vi "ZLIB Inflate__ogtk.vi"(4 "error in (no error)":errorcluster, 6 "expected length (try out)":i32, 7 "input":string) -> (0 "error out":errorcluster, 2 "length":i32, 3 "inflated output":string)   [LabVIEW 2014]
doc: "Inflates data previously deflated with ZLIB Deflate. \"input\" is the deflated data string and this vi returns the restored data in \"inflated output\". \nIn order to return the restored data a buffer needs to be allocated. The user of this routine should have stored the size of the original data outside of the compressed data and provide this size to the \"expected length\" input. Alternatively if the original size is unknown, leaving that parameter open will initially try with double the input buffer size and then retry 3 times each time doubling the buffer size again. This should work for data compressible up to 94%. Since a new buffer is allocated each time again and the data is decompressed into this buffer each time again, it is a good idea to actually provide the correct buffer size whenever possible to improve performance.\nThis VI uses the ZLIB compression routines.\n\nReturns \"Generic Error\" (42) when the zlib routine encountered any errors."
uses:
  <userlib>/_OpenG.lib/lvzip/lvzlib.dll
panel:
  # "Please visit http://www.OpenG.org to learn about the\nOpen Source LabVIEW software movement.\n\nNOTICE -- YOU MUST LEAVE THIS NOTICE IN PLACE.  PER THE TERMS OF THE LICENSE BELOW, YOU MAY SUBLICENSE THIS SOFTWARE \nIN ANY WAY THAT DOES NOT CONFLICT WITH THIS LICENSE.\n\n### BSD License (http://www.opensource.org/licenses/bsd-license.php) Begin ###\n \nCopyright (C) 2002 Rolf Kalbermatter rolf.kalbermatter@citeng.com\nCopyright (C) 2002 Jim Kring jim@jimkring.com\n\nAll rights reserved.\n\nRedistribution and use in source and binary forms, with or without modification, are permitted provided that the following conditions are met:\n\n    * Redistributions of source code must retain the above copyright notice, this list of conditions and the following disclaimer.\n    * Redistributions in binary form must reproduce the above copyright notice, this list of conditions and the following disclaimer in the \n       documentation and/or other materials provided with the distribution.\n    * Neither the name of SciWare, James Kring, Inc., nor the names of its contributors may be used to endorse or promote products derived \n       from this software without specific prior written permission.\n\nTHIS SOFTWARE IS PROVIDED BY THE COPYRIGHT HOLDERS AND CONTRIBUTORS \"AS IS\" AND ANY EXPRESS OR IMPLIED WARRANTIES, \nINCLUDING, BUT NOT LIMITED TO, THE IMPLIED WARRANTIES OF MERCHANTABILITY AND FITNESS FOR A PARTICULAR PURPOSE ARE \nDISCLAIMED. IN NO EVENT SHALL THE COPYRIGHT OWNER OR CONTRIBUTORS BE LIABLE FOR ANY DIRECT, INDIRECT, INCIDENTAL,\n SPECIAL, EXEMPLARY, OR CONSEQUENTIAL DAMAGES (INCLUDING, BUT NOT LIMITED TO, PROCUREMENT OF SUBSTITUTE GOODS OR \nSERVICES; LOSS OF USE, DATA, OR PROFITS; OR BUSINESS INTERRUPTION) HOWEVER CAUSED AND ON ANY THEORY OF LIABILITY, \nWHETHER IN CONTRACT, STRICT LIABILITY, OR TORT (INCLUDING NEGLIGENCE OR OTHERWISE) ARISING IN ANY WAY OUT OF THE USE \nOF THIS SOFTWARE, EVEN IF ADVISED OF THE POSSIBILITY OF SUCH DAMAGE.\n\n### BSD License End ###"
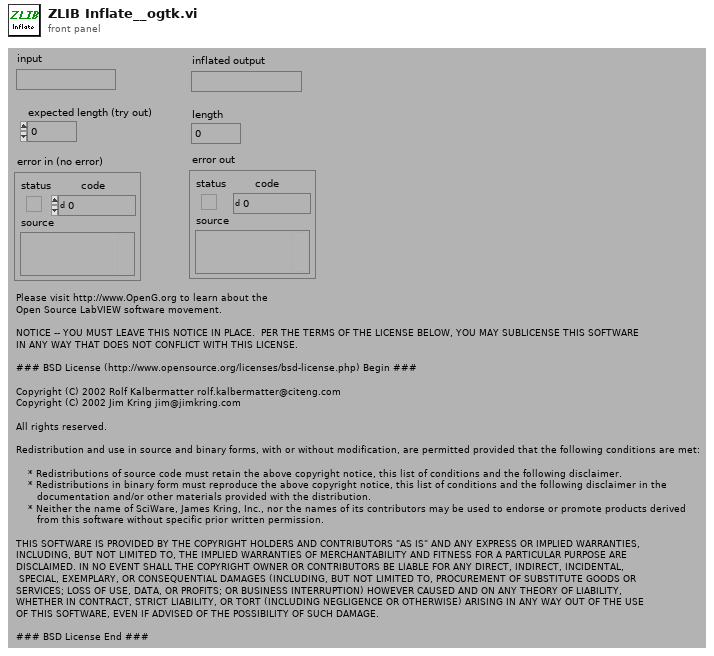
[diagram p1: front panel]
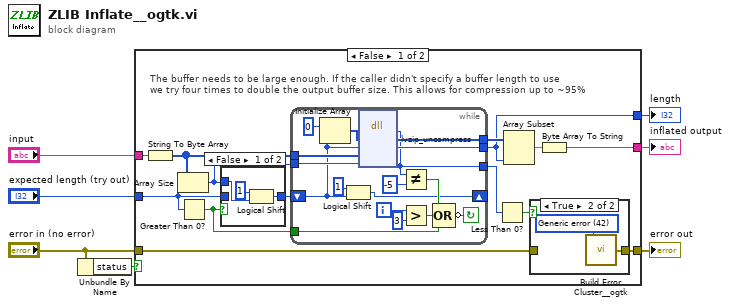
[diagram p0: block diagram]
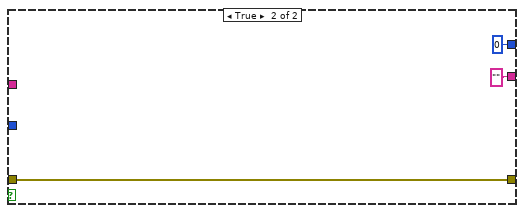
[diagram p4: hidden frame]
diagram:
  n1 = Unbundle By Name("error in (no error)") -> ("status"=w7:bool)
  n2 = case shown="False" w7 {
    tunnel: "error in (no error)" -> [w20 w48]
    tunnel: [w19 w48] -> w5
    tunnel: "input" -> [w18 _]
    tunnel: [w15 0 ("destLen")] -> w3
    tunnel: [w13 "" ("string")] -> w2
    tunnel: "expected length (try out)" -> [w12 _]
    frame False {
      # "The buffer needs to be large enough. If the caller didn't specify a buffer length to use\nwe try four times to double the output buffer size. This allows for compression up to ~95%"
      n3 = String To Byte Array(string=w18) -> (unsigned byte array=w17:u8[])
      n4 = Array Size(array=w17) -> (size(s)=w11:i32)
      n5 = Greater Than 0?(x=w12) -> (x > 0?=w9:bool)
      n6 = case shown="False" w9 {
        tunnel: w12 -> [_ w42]
        tunnel: w11 -> [w40 _]
        tunnel: [w39 w42] -> w10
        frame False {
          n7 = Logical Shift(y=1, x=w40) -> (x << y=w39:i32)
        }
        frame True {
        }
      }
      n8 = while {
        tunnel: w9 -> [w22]
        shift-left: w10 -> [w28]
        shift-right: [w26] -> _
        tunnel: w11 -> [w33]
        tunnel: [w36] -> w15
        tunnel: [w37] -> w16
        tunnel: w17 -> [w38]
        tunnel: [w32] -> w8
        i -> [w24]
        stop <- w29 continue-if-true
        n9 = Initialize Array(u8 0 ("Element Data"), w28) -> (w35:u8[])
        n10 = Logical Shift(y=1, x=w28) -> (x << y=w26:i32)
        n11 = dll-call lib="C:/Program Files (x86)/National Instruments/LabVIEW 2014/user.lib/_OpenG.lib/lvzip/lvzlib.*" fn="lvzip_uncompress"("pDest"=w35, "destLen"=w28, "pSource"=w38, "sourceLen"=w33) -> (w32:i32, "pDest"=w37:u8[], "destLen"=w36:i32)  [unwired: 5 in, 2 out]
        n12 = Not Equal?(x=w32, y=-5) -> (x != y?=w30:bool)
        n13 = Greater?(x=w24, y=3) -> (0:w25:bool)
        n14 = Compound Arithmetic op=OR(w30, w25, w22) -> (invert w29:bool)
      }
      n15 = Less Than 0?(x=w8) -> (x < 0?=w21:bool)
      n16 = Array Subset(array=w16, length=w15) -> (w14:u8[])  [unwired: 1 in]
      n17 = case shown="True" w21 {
        tunnel: [w43 w45] -> w19
        tunnel: w20 -> [w43 _]
        frame False {
        }
        frame True {
          w44 = 42 items=["No error", "Argument error", "Memory is full", "Out of zone", "End of file", "File already open", "Generic file I/O error", "File not found", "File permission error", "Disk is full", "Duplicate path", "Too many files open", "System feature not enabled", "Resource file not found", "Cannot add resource", "Resource not found", "Image not found", "Image memory error", "Pen does not exist", "Config type invalid", "Config token not found", "Config parse error", "Config memory error", "Bad external code format", "Bad external code offset", "External code not present", "Null window", "Destroy window error", "Null menu", "Print aborted", "Bad print record", "Print driver error", "Windows error during printing", "Memory error during printing", "Print dialog error", "Generic print error", "Invalid device refnum", "Device not found", "Device parameter error", "Device unit error", "Cannot open device", "Device call aborted", "Generic error", "Cancelled by user", "Object ID too low", "Object ID too high", "Object not in heap", "Unknown heap", "Unknown object (invalid DefProc)", "Unknown object (DefProc not in table)", "Message out of range", "Invalid (null) method", "Unknown message", "Manager call not supported", "Bad address", "Network operation in progress", "Network operation timed out", "Connection is busy", "Network attribute not supported", "Network error", "Address in use", "System out of memory", "Connection aborted", "Connection refused", "Not connected", "Already connected", "Connection closed", "Initialization error (interapplication manager)", "Bad occurrence", "Wait on unbound occurrence handler", "Occurrence queue overflow", "Datalog type conflict", "Unused", "Unrecognized type (interapplication manager)", "Memory corrupt", "Failed to make temporary DLL", "Old CIN version", "Drag socket not found", "Failed to load drop-object", "Failed to register OLE object", "Failed to release OLE object", "Format specifier type mismatch", "Unknown format specifier", "Too few format specifiers", "Too many format specifiers", "Scan failed", "Newer CIN version", "Error converting to variant", "Runtime menu error", "Password tampered", "Variant attribute not found", "Incompatible variant data type", "Event data is not available", "Event Store is not present", "Occurrence is not found", "Event Queue is not created", "Event info is not available", "Refnum passed is NULL", "Error retrieving Class GUID", "Error retrieving CoClass GUID", "Error retrieving TypeLib GUID.", "Bad built application magic bytes.", "Specific driver is different from the specific driver associated with the Logical Name.", "There is no session opened to the class driver.", "Max Error", "MAX - Error with config objects", "MAX - Error loading configuration", "MAX - Group not supported"]
          n18 = call <userlib>:"Build Error Cluster__ogtk.vi"("code"=w44) -> ("error out"=w45:errorcluster)  [unwired: 1 in]
        }
      }
      n19 = Byte Array To String(unsigned byte array=w14) -> (string=w13:string)
    }
    frame True {
    }
  }
  "error out" <- w5
  "inflated output" <- w2
  "length" <- w3
